vi "Extract Anthropic Response.vi"(0 "headers":string, 5 "body":string, 11 "error in":errorcluster) -> (4 "value":string, 15 "error out":errorcluster)   [LabVIEW 2020, in "llm_anthropic_chatmodels.lvclass"]
uses:
  llm_anthropic_chatmodels.lvclass
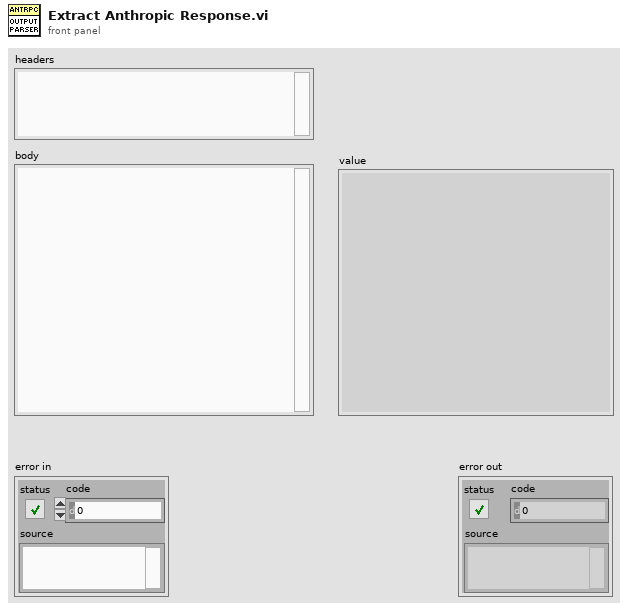
[diagram p1: front panel]
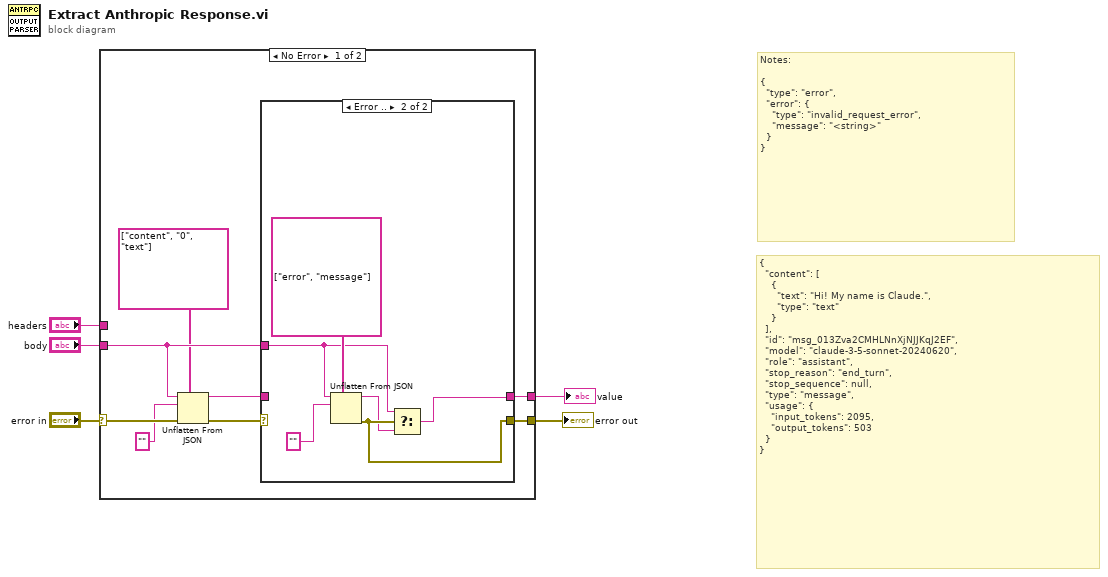
[diagram p0: block diagram]
diagram:
  # "{\n  \"content\": [\n    {\n      \"text\": \"Hi! My name is Claude.\",\n      \"type\": \"text\"\n    }\n  ],\n  \"id\": \"msg_013Zva2CMHLNnXjNJJKqJ2EF\",\n  \"model\": \"claude-3-5-sonnet-20240620\",\n  \"role\": \"assistant\",\n  \"stop_reason\": \"end_turn\",\n  \"stop_sequence\": null,\n  \"type\": \"message\",\n  \"usage\": {\n    \"input_tokens\": 2095,\n    \"output_tokens\": 503\n  }\n}"
  # "Notes:\n\n{\n  \"type\": \"error\",\n  \"error\": {\n    \"type\": \"invalid_request_error\",\n    \"message\": \"<string>\"\n  }\n}"
  n1 = case shown="No Error" "error in" {
    selector: "error in" -> [w13 w23]
    tunnel: [w10 w23] -> w4
    tunnel: "body" -> [w9 _]
    tunnel: "headers" -> [_ w22]
    tunnel: [w7 w22] -> w1
    frame No Error {
      n2 = Unflatten From JSON(path=string[] ["content", "0", "text"], JSON string=w9, type and defaults="", error in (no error)=w13) -> (value=w8:string, error out=w11:errorcluster)  [unwired: 3 in]
      n3 = case shown="Error .." w11 {
        selector: w11 -> [w15 _]
        tunnel: [w15 w18] -> w10
        tunnel: w9 -> [_ w16]
        tunnel: w8 -> [w14 _]
        tunnel: [w14 w19] -> w7
        frame No Error {
        }
        frame Error {
          n4 = Unflatten From JSON(path=string[] ["error", "message"], JSON string=w16, type and defaults="") -> (value=w17:string, error out=w18:errorcluster)  [unwired: 4 in]
          n5 = Select(t=w16, s=w18, f=w17) -> (s? t:f=w19:string)
        }
      }
    }
    frame Error {
    }
  }
  "error out" <- w4
  "value" <- w1
